vi "Get Output.vi"(8 "error in (no error)":errorcluster, 11 "Command Execution in":refnum<class "Command Execution.lvclass">) -> (0 "error out":errorcluster, 2 "Output":string, 3 "Command Execution out":refnum<class "Command Execution.lvclass">)   [LabVIEW 2015, in "WinSCP.lvlib" / "Command Execution.lvclass"]
uses:
  Command Execution.lvclass
  Command Execution.lvclass/Command Execution.ctl
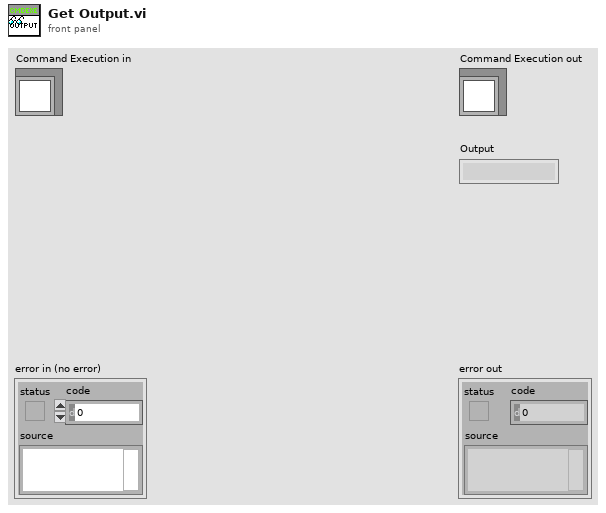
[diagram p1: front panel]
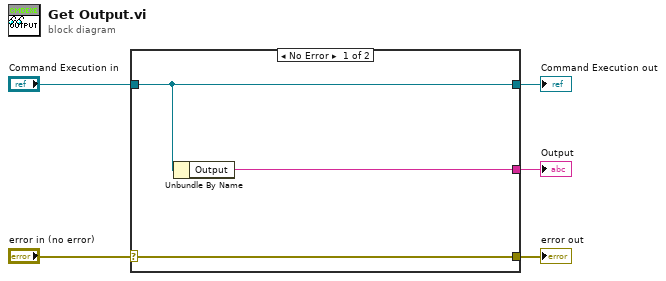
[diagram p0: block diagram]
diagram:
  n1 = case shown="No Error" "error in (no error)" {
    selector: "error in (no error)" -> [w8 w9]
    tunnel: [w8 w9] -> w4
    tunnel: [w7 w10] -> w2
    tunnel: "Command Execution in" -> [w7 w10]
    tunnel: [w6 _] -> w1
    frame No Error {
      n2 = Unbundle By Name(w7) -> ("Output"=w6:string)
    }
    frame Error {
    }
  }
  "error out" <- w4
  "Command Execution out" <- w2
  "Output" <- w1
